vi "Start Experiment.vi"(8 "error in (no error)":errorcluster, 10 "Memory":bool=TRUE, 11 "Pulseblaster in":refnum<class "Pulseblaster.lvclass">) -> (0 "error out":errorcluster, 3 "Pulseblaster out":refnum<class "Pulseblaster.lvclass">)   [LabVIEW 2013, in "Pulseblaster.lvclass"]
uses:
  Pulseblaster.lvclass
  Utils_devs/SpinAPI/SpinAPI-Interface.lvlib
panel:
  # "SOFTWARE TRIGGER"
  # "External"
  # "Internal"
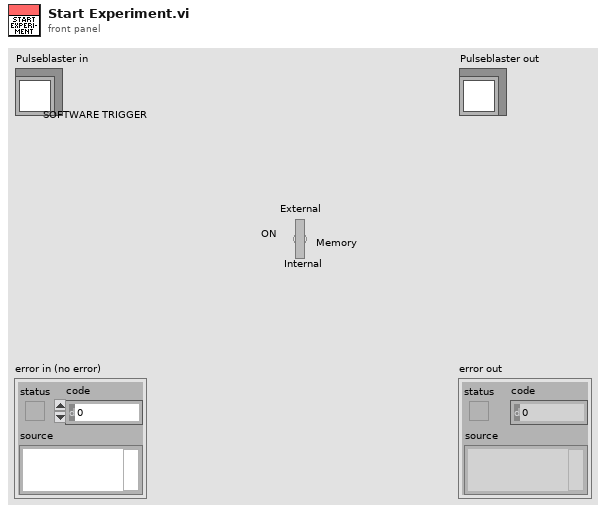
[diagram p1: front panel]
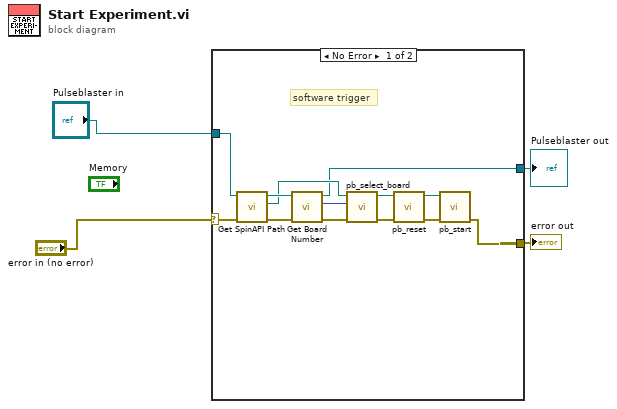
[diagram p0: block diagram]
diagram:
  n1 = case shown="No Error" "error in (no error)" {
    selector: "error in (no error)" -> [w10 w19]
    tunnel: [w9 w19] -> w3
    tunnel: "Pulseblaster in" -> [w12 w18]
    tunnel: [w11 w18] -> w1
    frame No Error {
      # "software trigger"
      n2 = call-dynamic "Get SpinAPI Path.vi"("error in (no error)"=w10, "Pulseblaster in"=w12) -> ("error out"=w17:errorcluster, "SpinAPI Path"=w13:path, "Pulseblaster out"=w14:refnum<class "Pulseblaster.lvclass">)  [unwired: 7 in]
      n3 = call-dynamic "Get Board Number.vi"("error in (no error)"=w17, "Pulseblaster in"=w14) -> ("error out"=w16:errorcluster, "Board Number"=w15:i32, "Pulseblaster out"=w11:refnum<class "Pulseblaster.lvclass">)  [unwired: 7 in]
      n4 = call "pb_select_board.vi"("error in (no error)"=w16, "board_num"=w15, "path in"=w13) -> ("error out"=w8:errorcluster, "path out"=w5:path)  [unwired: 7 in]
      n5 = call "pb_reset.vi"("error in (no error)"=w8, "path in"=w5) -> ("error out"=w7:errorcluster, "path out"=w6:path)  [unwired: 8 in]
      n6 = call "pb_start.vi"("error in (no error)"=w7, "path in"=w6) -> ("error out"=w9:errorcluster)  [unwired: 8 in, 1 out]
    }
    frame Error {
    }
  }
  "error out" <- w3
  "Pulseblaster out" <- w1
